vi "PL_estimator.vi"(11 "measured_signal":T1) -> (0 "quality_check":bool, 2 "fit_parameters":T3 {"mse" format="%#_3e"; "Tb" format="%.3g"; "B" format="%.3g"; "Ta" format="%.3g"; "A" format="%.3g"; "Ie" format="%.3g"}, 3 "fitted_signal":T2)   [LabVIEW 2018]
uses:
  <vilib>/Analysis/6fits.llb/Curve Fitting Criteria.ctl
  <vilib>/gmath/NumericalOptimization/Nonlinear Curve Fit LM bound.vi
  <vilib>/gmath/NI_Gmath.lvlib
  <vilib>/Analysis/NI_AALPro.lvlib
panel:
  out "XY Graph":T4(graph)
  # "Photoluminescence signal model:"
  # "I(t) = I(inf) + A * exp(-t/Ta) + B * exp(-t/Tb)]"
  # "T1 := max(Ta, Tb)"
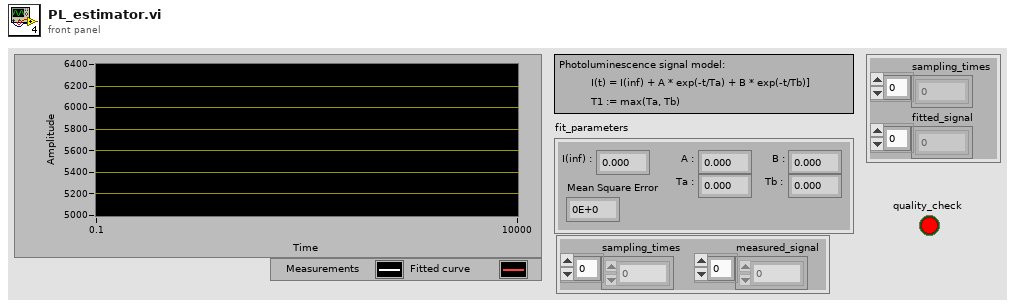
[diagram p1: front panel]
types:
  T1 = cluster{"sampling_times":dbl[], "measured_signal":dbl[]}
  T2 = cluster{"sampling_times":dbl[], "fitted_signal":dbl[]}
  T3 = cluster{"Ie":dbl, "A":dbl, "Ta":dbl, "B":dbl, "Tb":dbl, "mse":dbl}
  T4 = cluster{"log_samples_us":dbl[], "best nonlinear fit":dbl[]}[]
  T5 = cluster{"parameter minimum":dbl[], "parameter maximum":dbl[]}
  T6 = typedef "NI_AALPro.lvlib/Curve Fitting Criteria.ctl" = u16
  T7 = cluster{"sampling_times":dbl[], "best nonlinear fit":dbl[]}
  T8 = cluster{"sampling_times":dbl[], "best nonlinear fit":dbl[]}[]
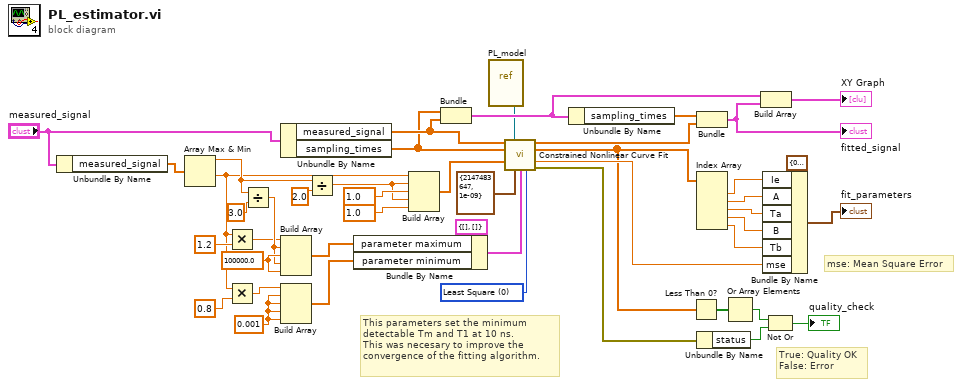
[diagram p0: block diagram]
diagram:
  w6 = 0.001 ("element")
  w15 = 100000.0 ("element")
  w31 = T6 0 items=["Least Square", "Least Absolute Residual", "Bisquare"] ("method")
  # "This parameters set the minimum \ndetectable Tm and T1 at 10 ns.\nThis was necesary to improve the\nconvergence of the fitting algorithm."
  # "True: Quality OK\nFalse: Error"
  # "mse: Mean Square Error"
  n1 = Unbundle By Name("measured_signal") -> ("measured_signal"=w18:dbl[])
  n2 = Array Max & Min(array=w18) -> (max value=w8:dbl, min value=w2:dbl)  [unwired: 2 out]
  n3 = Multiply(x=w2, y=1.2 ("x")) -> (x*y=w1:dbl)
  n4 = Multiply(x=w2, y=0.8 ("x")) -> (x*y=w4:dbl)
  n5 = Divide(x=w8, y=3.0) -> (x/y=w9:dbl)
  n6 = Unbundle By Name("measured_signal") -> ("measured_signal"=w37:dbl[], "sampling_times"=w36:dbl[])
  n7 = Build Array(w1, w9, w15, w9, w15) -> (w17:dbl[])
  n8 = Build Array(w4, w6, w6, w6, w6) -> (w16:dbl[])
  n9 = Divide(x=w8, y=2.0) -> (x/y=w11:dbl)
  n10 = Bundle By Name(cluster=T5 {"parameter minimum"=[], "parameter maximum"=[]} ("parameter bounds"), "parameter maximum"=w17, "parameter minimum"=w16) -> (w29:T5)
  n11 = Build Array(w2, w11, 1.0 ("element"), w11, 1.0 ("element")) -> (w14:dbl[])
  n12 = Bundle("sampling_times"=w36, "measured_signal"=w37) -> (w44:T1)  [unwired: 1 in]
  n13 = vi-ref "PL_model.vi"() -> (w33:refnum<vi>)
  n14 = call-poly <vilib>:"Constrained Nonlinear Curve Fit.vi"("Y"=w37, "f(x,a)"=w33, "X"=w36, "initial parameters"=w14, "termination"=cluster{"max iteration":i32, "tolerance":dbl} {"max iteration"=2147483647, "tolerance"=1e-09}, "parameter bounds"=w29, "method"=w31) -> ("best nonlinear fit"=w34:dbl[], "best fit parameters"=w21:dbl[], "residue"=w22:dbl, "error out"=w35:errorcluster)  [unwired: 3 in, 2 out]
  n15 = Unbundle By Name(w44) -> ("sampling_times"=w42:dbl[])
  n16 = Less Than 0?(x=w21) -> (x < 0?=w41:bool[])
  n17 = Bundle("sampling_times"=w42, "best nonlinear fit"=w34) -> (w45:T7)  [unwired: 1 in]
  "fitted_signal" <- w45
  n18 = Index Array(array=w21) -> (element #1=w27:dbl, element #2=w26:dbl, element #3=w25:dbl, element #4=w24:dbl, element #5=w23:dbl)  [unwired: 5 in]
  n19 = Unbundle By Name(w35) -> ("status"=w39:bool)
  n20 = Or Array Elements(Boolean array=w41) -> (logical OR=w40:bool)
  n21 = Build Array(w44, w45) -> (→"XY Graph":T8)
  n22 = Bundle By Name(cluster=T3 {"Ie"=0.0, "A"=0.0, "Ta"=0.0, "B"=0.0, "Tb"=0.0, "mse"=0.0} ("fit_parameters"), "Ie"=w27, "A"=w26, "Ta"=w25, "B"=w24, "Tb"=w23, "mse"=w22) -> (→"fit_parameters":T3)
  n23 = Not Or(1:w39, 2:w40) -> (0:→"quality_check":bool)
